vi "Read Class from Error.vi"(8 "Error in":errorcluster) -> (0 "Error out":errorcluster, 2 "Class Detected":bool, 3 "Class":string)   [LabVIEW 2019, in "Logger.Error.lvlib" / "Logger.Error.lvclass"]
doc: "This VI returns and removes \"classification\" information that was previously attached to an error using the Classify Error VI or the Specific Error Handler. This VI is typically called as part of a Central Error Handler. This VI modifies the source string of the error to remove the classification."
uses:
  Logger.Error.lvclass
  <vilib>/regexp/Match Regular Expression.xnode
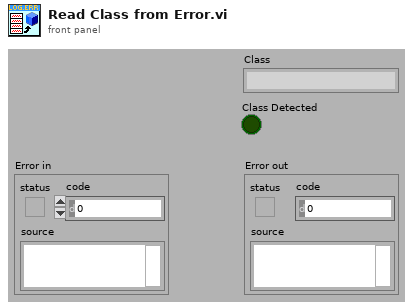
[diagram p1: front panel]
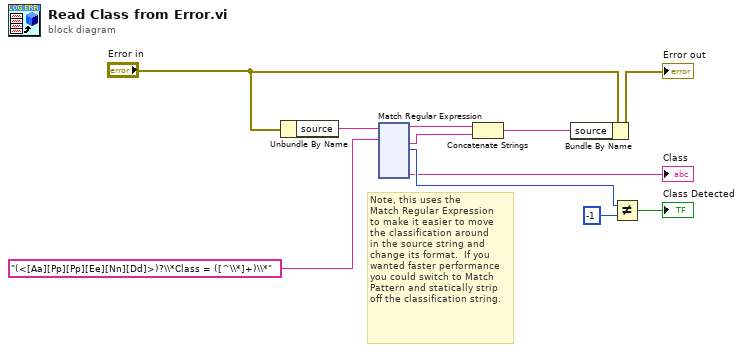
[diagram p0: block diagram]
diagram:
  # "Note, this uses the\nMatch Regular Expression\nto make it easier to move\nthe classification around\nin the source string and\nchange its format.  If you\nwanted faster performance\nyou could switch to Match\nPattern and statically strip\noff the classification string."
  n1 = Unbundle By Name("Error in") -> ("source"=w7:string)
  n2 = xnode "Match Regular Expression"("input string"=w7, "regular expression"="(<[Aa][Pp][Pp][Ee][Nn][Dd]>)?\\*Class = ([^\\*]+)\\*" ("regular expression (\"\")")) -> ("before match"=w6:string, "after match"=w5:string, "offset past match"=w4:i32, "submatch 2"=→"Class":string)  [unwired: 2 in, 5 out]
  n3 = Concatenate Strings(w6, w5) -> (w9:string)
  n4 = Bundle By Name(cluster="Error in", "source"=w9) -> (→"Error out":errorcluster)
  n5 = Not Equal?(x=w4, y=-1) -> (x != y?=→"Class Detected":bool)
